vi "dfd_Get Matrix U.vi"(6 "para":dbl, 8 "error in (no error)":errorcluster, 9 "order":i32, 10 "number of bans":i32, 11 "half h":dbl[](array[numeric])) -> (0 "error out":errorcluster, 3 "U":dbl[][](array[numeric]))   [LabVIEW 2017, in "NI_DigFilter_FilterBank.lvlib"]
uses:
  <vilib>/addons/Digital Filter Design/NI_DigFilter_FilterBank.lvlib
  <vilib>/Analysis/baseanly.llb/Real A x B.vi
  <vilib>/addons/Digital Filter Design/_Misc.llb/dfd_Error Cluster From Error Code (Scalar).vi
  <vilib>/addons/Digital Filter Design/_LpNorm.llb/dfd_Left Multiply Diagonal Matrix (Real).vi
  <vilib>/Analysis/NI_AALBase.lvlib
  <vilib>/addons/Digital Filter Design/NI_DigFilterLicensed.lvlib
  <vilib>/addons/Digital Filter Design/NI_DigFilter_Design.lvlib
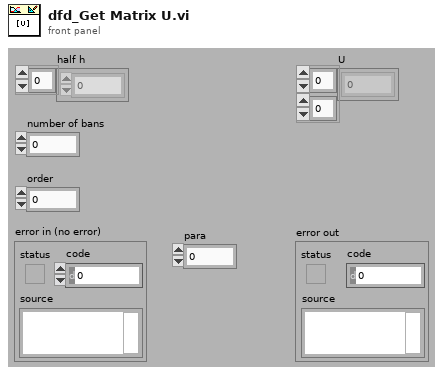
[diagram p1: front panel]
types:
  T1 = typedef "NI_Matrix.lvlib/RealMatrix.ctl" = dbl[][]
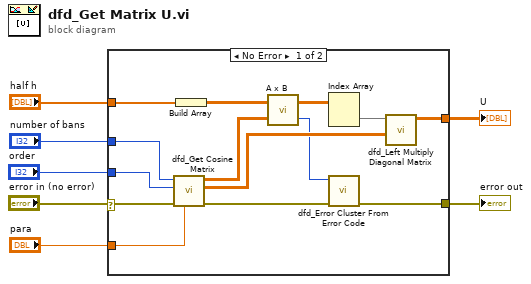
[diagram p0: block diagram]
diagram:
  n1 = case shown="No Error" "error in (no error)" {
    selector: "error in (no error)" -> [w9 w22]
    tunnel: "number of bans" -> [w21 _]
    tunnel: "half h" -> [w8 _]
    tunnel: [w19 _] -> w5
    tunnel: "para" -> [w17 _]
    tunnel: "order" -> [w13 _]
    tunnel: [w10 w22] -> w2
    frame No Error {
      n2 = call <vilib>:"dfd_Get Cosine Matrix.vi"("w"=w17, "error in (no error)"=w9, "order"=w13, "number of bands"=w21) -> ("error out"=w11:errorcluster, "CT"=w14:dbl[][], "C"=w18:dbl[][])  [unwired: 5 in]
      n3 = Build Array(w8) -> (w20:dbl[][])
      n4 = call-poly <vilib>:"A x B.vi"("B"=w18, "A"=w20) -> ("error"=w12:i32, "A x B"=w16:T1)
      n5 = Index Array(array=w16) -> (element=w15:dbl[])  [unwired: 2 in]
      n6 = call-poly <vilib>:"dfd_Error Cluster From Error Code.vi"("error in (no error)"=w11, "error code (0)"=w12) -> ("error out"=w10:errorcluster)  [unwired: 9 in]
      n7 = call-poly <vilib>:"dfd_Left Multiply Diagonal Matrix.vi"("B"=w14, "diagonal"=w15) -> ("diagonal x B"=w19:dbl[][])  [unwired: 8 in, 1 out]
    }
    frame Error {
    }
  }
  "U" <- w5
  "error out" <- w2
